vi "FRCts20_Backend_TeamRoot_PPD_reform.vi"(7 "Team Root":T1, 8 "error in (no error)":errorcluster, 11 "rows affected":i32) -> (0 "error out":errorcluster, 2 "data string":string)   [LabVIEW 2014, in "FRCts20_Backend_Engine.lvlib"]
doc: "Returns whether a new team was successfully created"
uses:
  FRCts20_Backend_Engine.lvlib
  FRCts20_Backend_API/FRCts20_Backend_API_TeamRoot.ctl
  FRCts20_Backend_API/FRCts20_Backend_API_SW.ctl
  FRCts20_Backend_API/FRCts20_Backend_API.lvlib
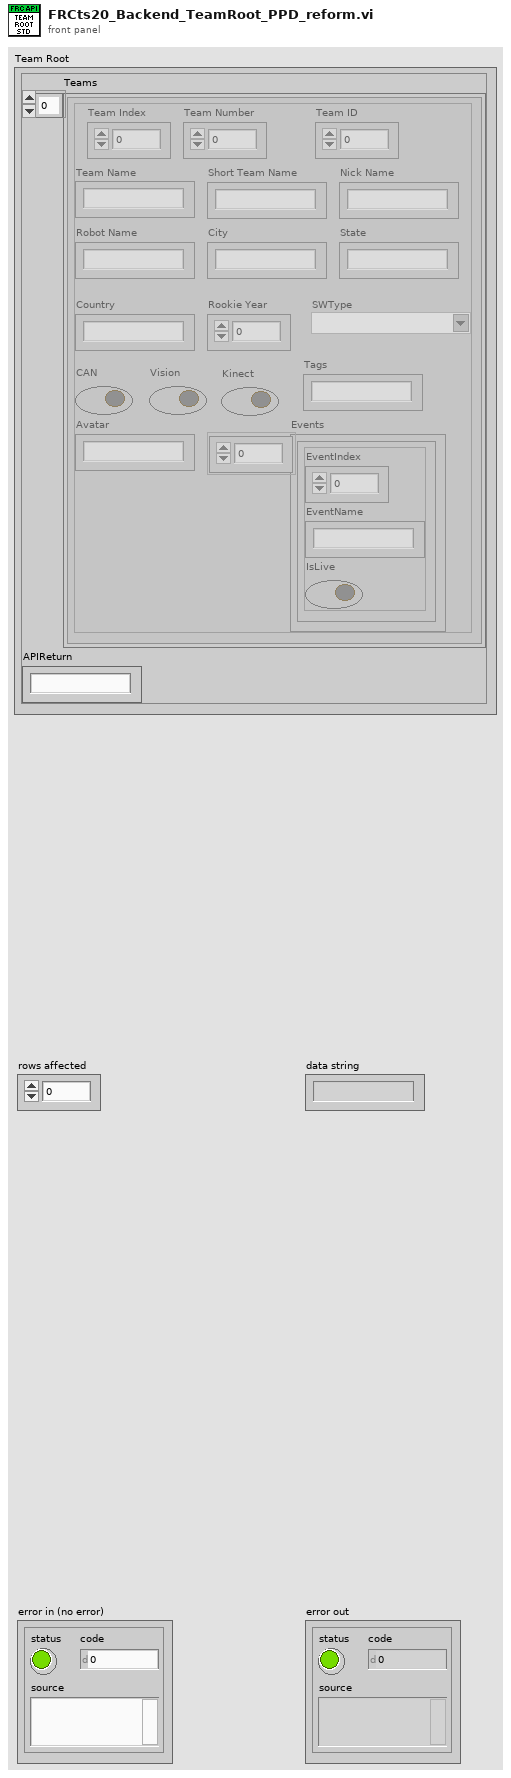
[diagram p1: front panel]
types:
  T1 = typedef "FRCts20_Backend_API.lvlib/FRCts20_Backend_API_TeamRoot.ctl" = cluster{"Teams":cluster{"Team Index":u32, "Team Number":u32, "Team ID":u32, "Team Name":string, "Short Team Name":string, "Nick Name":string, "Robot Name":string, "City":string, "State":string, "Country":string, "Rookie Year":u32, "SWType":T2, "CAN":bool, "Vision":bool, "Kinect":bool, "Tags":string, "Avatar":string, "Events":cluster{"EventIndex":u32, "EventName":string, "IsLive":bool}[]}[], "APIReturn":string}
  T2 = typedef "FRCts20_Backend_API.lvlib/FRCts20_Backend_API_SW.ctl" = string
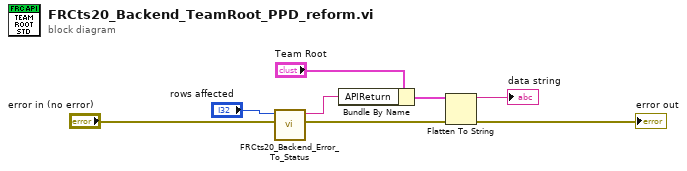
[diagram p0: block diagram]
diagram:
  n1 = call "FRCts20_Backend_Error_To_Status.vi"("error in (no error)"="error in (no error)", "rows affected"="rows affected") -> ("error out"=w4:errorcluster, "String"=w5:string)  [unwired: 8 in]
  n2 = Bundle By Name(cluster="Team Root", "APIReturn"=w5) -> (w1:T1)
  n3 = Flatten To String(anything=w1, error in (no error)=w4) -> (data string=→"data string":string, error out=→"error out":errorcluster)  [unwired: 2 in, 1 out]
